vi "Query with Result_test.vi"(7 "UserName":string="Jimbo", 8 "error in (no error)":errorcluster, 10 "Search Parameters":T2[](array[typedef])=[{"eSearch Types"=enum."eSearchFile", "Property Name"="registertxt2", "DataFinder Comparisons"=enum."=", "Property Value"="*"}], 11 "eSearch Type":T1=enum."eSearchChannelGroup") -> (0 "error out":errorcluster={"status"=FALSE, "code"=2552, "source"="_createExplicitChildObject.vi"}, 1 "Result TDM":path, 2 "Number of Items":i32, 3 "Results":string[][](array[string]), 4 "Data Returned?":bool)   [LabVIEW 2011]
uses:
  eSearch Types.ctl
  DataFinder Comparisons.ctl
  Datafinder Query.ctl
panel:
  in  "Case Constant\n(See Context Help)":bool=TRUE
  # "The query passes back an array of [ Filepath, MN, SN, RunID, CHID, Cond1, ... CondN] per row."
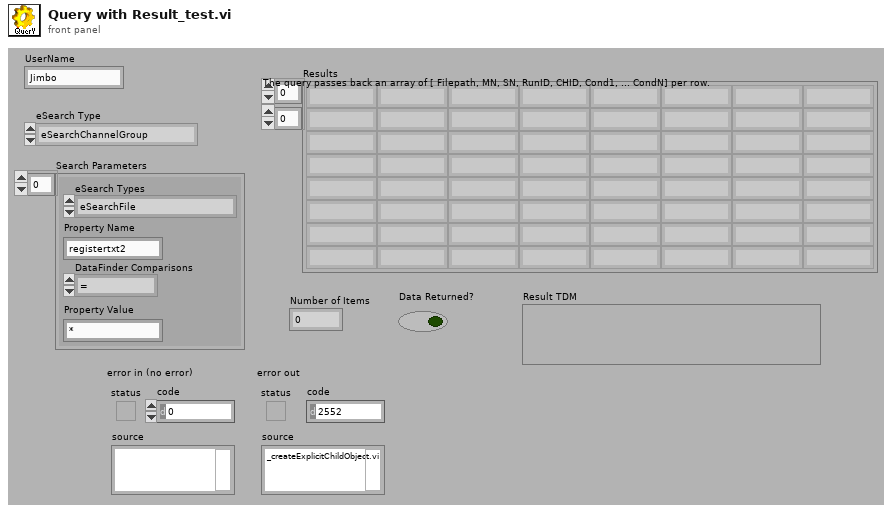
[diagram p1: front panel]
types:
  T1 = typedef "eSearch Types.ctl" = enum16{"eSearchFile", "eSearchChannelGroup", "eSearchChannel"}
  T2 = typedef "Datafinder Query.ctl" = cluster{"eSearch Types":T1, "Property Name":string, "DataFinder Comparisons":T3, "Property Value":string}
  T3 = typedef "DataFinder Comparisons.ctl" = enum16{"=", "<>", "<", "<=", ">", ">="}
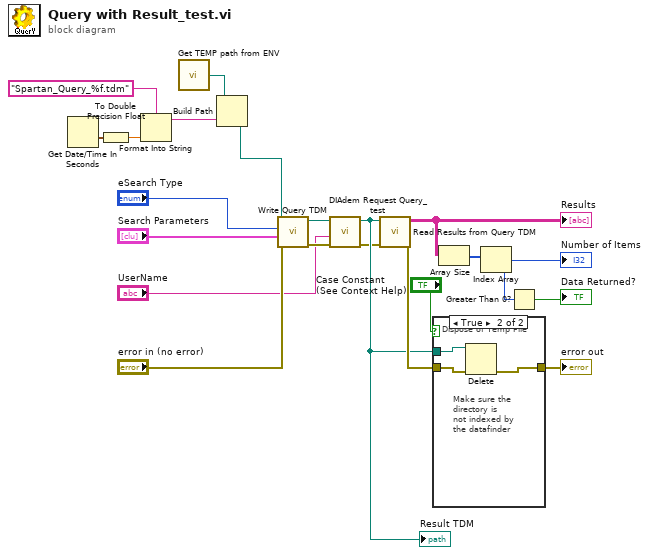
[diagram p0: block diagram]
diagram:
  n1 = Get Date/Time In Seconds() -> (seconds since 1Jan1904=w15:timestamp)
  n2 = To Double Precision Float(number=w15) -> (double precision float=w14:dbl)
  n3 = Format Into String(format string="Spartan_Query_%f.tdm", w14) -> (resulting string=w7:string)  [unwired: 2 in, 1 out]
  n4 = call "Get TEMP path from ENV.vi"() -> ("TEMP Path"=w8:path)  [unwired: 5 in]
  n5 = Build Path(base path=w8, name or relative path=w7) -> (appended path=w6:path)
  n6 = call "Write Query TDM.vi"("error in (no error)"="error in (no error)", "DataFinder parameters"="Search Parameters", "Return Type (ChannelGroup)"="eSearch Type", "Query Path"=w6) -> ("error out"=w4:errorcluster, "Query Path Out"=w5:path)  [unwired: 6 in]
  n7 = call "DIAdem Request Query_test.vi"("error in (no error)"=w4, "Username (empty)"="UserName", "Query TDM"=w5) -> ("error out"=w1:errorcluster, "Generated Report Path"=w2:path)  [unwired: 7 in]
  "Result TDM" <- w2
  n8 = call "Read Results from Query TDM.vi"("error in (no error)"=w1, "Query Path"=w2) -> ("error out"=w11:errorcluster, "Results"=w18:string[][])  [unwired: 8 in]
  "Results" <- w18
  n9 = case shown="True" "Case Constant\n(See Context Help)" {
    tunnel: w11 -> [w22 w25]
    tunnel: [w22 w24] -> w10
    tunnel: w2 -> [_ w23]
    frame False {
      # "8 error on\ndelete of TDM\nwait for NI to\nrespond\nor\nsometimes file\nis not deleted\nand .log file found"
    }
    frame True {
      # "Make sure the\ndirectory is \nnot indexed by\nthe datafinder"
      # "Dispose of Temp File"
      n10 = Delete(path (use dialog)=w23, error in=w25) -> (error out=w24:errorcluster)  [unwired: 3 in, 2 out]
    }
  }
  "error out" <- w10
  n11 = Array Size(array=w18) -> (size(s)=w17:i32[])
  n12 = Index Array(array=w17) -> (element=w13:i32)  [unwired: 1 in]
  "Number of Items" <- w13
  n13 = Greater Than 0?(x=w13) -> (x > 0?=→"Data Returned?":bool)
